vi "Examples.vi"(6 "Python version":string="3.9", 7 "Python":T1, 11 "Port":string) -> ()   [LabVIEW 2022 SP3]
uses:
  PythonCtrl.ctl
  Processors.ctl
panel:
  out "Python files":string[](array[string])
  in  "Location":bool
  in  "Folder":u16(ring) items=["home"]
  in  "Files":i32(listbox)
  in  "Code":string="Loading..."
  in  "Remove Button":bool
  in  "Paste":bool
  in  "Update":bool
  # "File Explorer\nversion 0"
  # "https://lego.github.io/MINDSTORMS-Robot-Inventor-hub-API/index.html"
  # "SPIKE Prime"
  # "Examples"
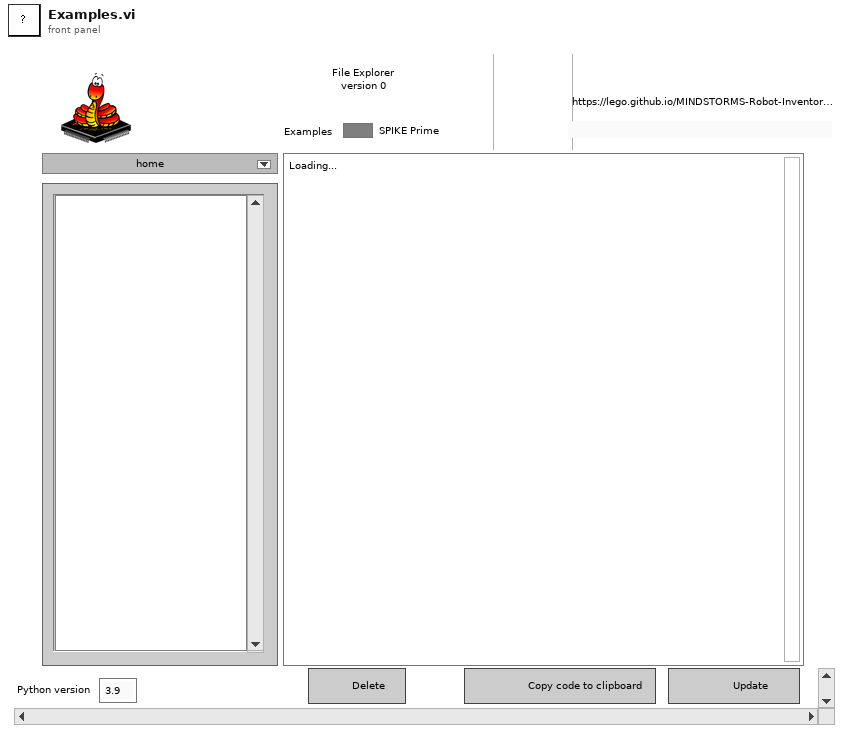
[diagram p1: front panel]
types:
  T1 = typedef "PythonCtrl.ctl" = cluster{"session":refnum<k35>, "PyPath":path, "Processor":T2, "Port":string, "version":string}
  T2 = typedef "Processors.ctl" = enum16{"SPIKE", "Pi", "Pi_ssh", "OpenMV", "Dunio"}
  T3 = enum16{"read", "write pause", "write port", "write path", "write all"}
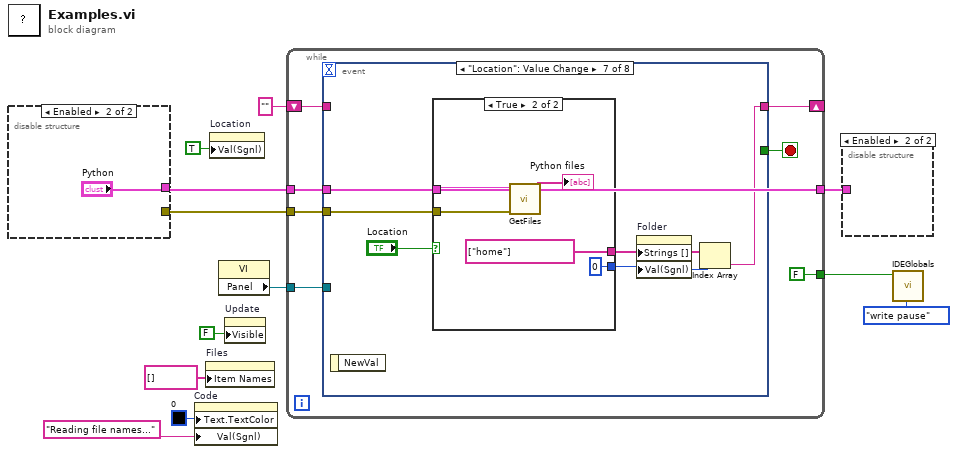
[diagram p0: block diagram]
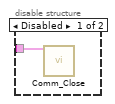
[diagram p2: hidden frame]
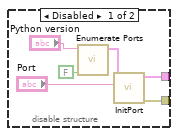
[diagram p3: hidden frame]
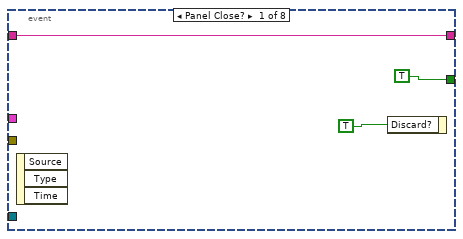
[diagram p4: hidden frame]
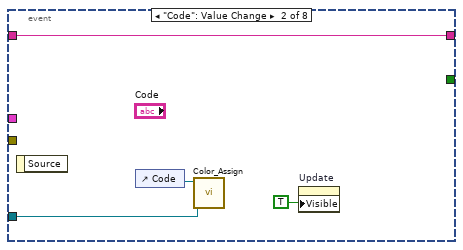
[diagram p5: hidden frame]
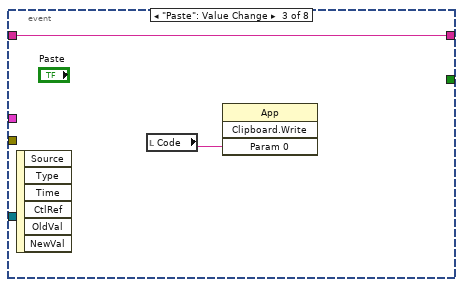
[diagram p6: hidden frame]
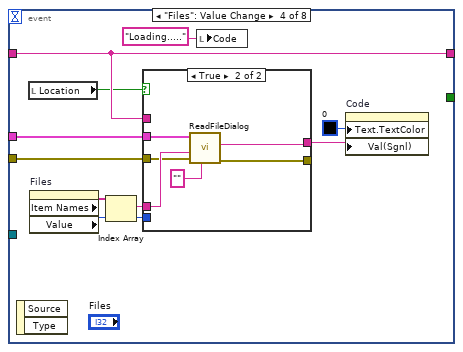
[diagram p7: hidden frame]
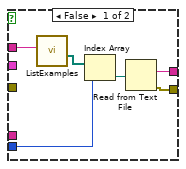
[diagram p8: hidden frame]
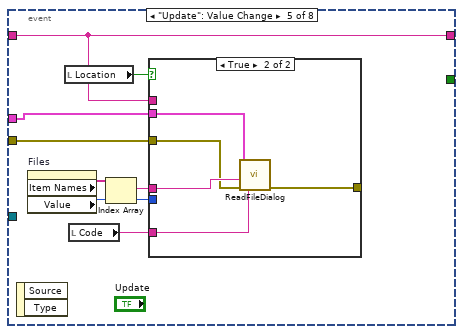
[diagram p9: hidden frame]
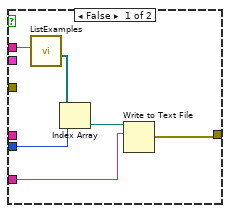
[diagram p10: hidden frame]
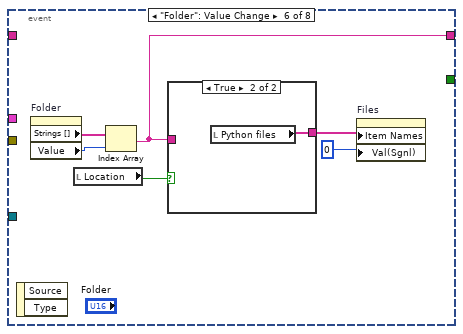
[diagram p11: hidden frame]
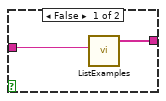
[diagram p12: hidden frame]
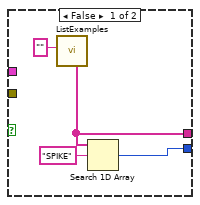
[diagram p13: hidden frame]
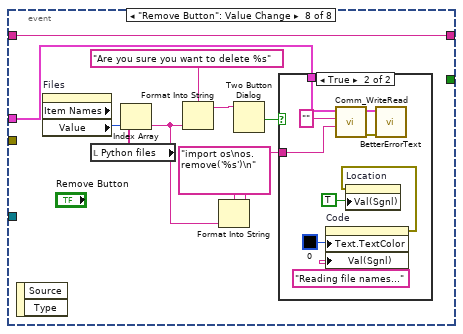
[diagram p14: hidden frame]
diagram:
  n1 = disable-structure shown="Enabled" {
    disable-tunnel: [w18 _] -> w7
    disable-tunnel: [w17 "Python"] -> w6
    frame Disabled {
      n2 = call "Enumerate Ports.vi"("list?"=FALSE, "Python version"="Python version") -> ("Python"=w15:T1)  [unwired: 4 in, 5 out]
      n3 = call "InitPort.vi"("Port"="Port", "Python"=w15) -> ("error out"=w18:errorcluster, "Python out"=w17:T1)  [unwired: 7 in, 1 out]
    }
    frame Enabled {
    }
  }
  n4 = property on="Code" class="Str"("Text.TextColor"=u32 0 ("Text.Text Colors:Text Color"), "Val(Sgnl)"="Reading file names...") -> ()  [unwired: 2 in, 2 out]
  n5 = property on="Files" class="LstBox (strict)"("Item Names"=string[] []) -> ()  [unwired: 2 in, 2 out]
  n6 = property on="Location" class="Bool (strict)"("Val(Sgnl)"=TRUE ("Value (Signaling)")) -> ()  [unwired: 2 in, 2 out]
  n7 = property class="VI"() -> ("Panel"=w12:refnum<vi>)  [unwired: 2 in, 2 out]
  n8 = property on="Update" class="Bool"("Visible"=FALSE) -> ()  [unwired: 2 in, 2 out]
  n9 = while {
    tunnel: w12 -> [w25]
    shift-right: [w24] -> _
    shift-left: "" ("Folder") -> [w23]
    tunnel: w6 -> [w20]
    tunnel: [FALSE ("pause?")] -> w1
    tunnel: w7 -> [w21]
    tunnel: [w20] -> w5
    stop <- w26 stop-if-true
    n10 = event shown="[6] \"Location\": Value Change" {
      selector: _ -> [_ _ _ _ _ _ _ _]
      dyn-events: _ -> [_ _ _ _ _ _ _ _]
      timeout: _ -> [_ _ _ _ _ _ _ _]
      tunnel: [TRUE ("stop") _ _ _ _ _ _ _] -> w26
      tunnel: w25 -> [_ w31 _ _ _ _ _ _]
      tunnel: [w27 w33 w35 w45 w65 w78 w89 w110] -> w24
      tunnel: w23 -> [w27 w33 w35 w45 w65 _ _ w110]
      tunnel: w20 -> [_ _ _ w43 w63 _ w91 w104]
      tunnel: w21 -> [_ _ _ w38 w58 _ w86 _]
      event Panel Close? {
        n11 = event-data() -> ()  [unwired: 1 in, 3 out]
        n12 = event-data("Discard?"=TRUE ("stop")) -> ()  [unwired: 1 in, 1 out]
      }
      event "Code": Value Change {
        n13 = event-data() -> ()  [unwired: 1 in, 1 out]
        n14 = control-ref of="Code"() -> (w30:refnum<vi>)
        n15 = call "Color_Assign.vi"("Front Panel"=w31, "Code"=w30) -> ()  [unwired: 9 in, 1 out]
        n16 = property on="Update" class="Bool"("Visible"=TRUE) -> ()  [unwired: 2 in, 2 out]
      }
      event "Paste": Value Change {
        n17 = event-data() -> ()  [unwired: 1 in, 6 out]
        n18 = local read "Code"() -> (w34:string)
        n19 = invoke class="App" method="Clipboard.Write"("Param 0"=w34) -> ()  [unwired: 3 in, 4 out]
      }
      event "Files": Value Change {
        n20 = event-data() -> ()  [unwired: 1 in, 2 out]
        n21 = local read "Location"() -> (w44:bool)
        n22 = property on="Files" class="LstBox (strict)"() -> ("Item Names"=w42:string[], "Value"=w40:i32)  [unwired: 2 in, 2 out]
        n23 = Index Array(array=w42, index=w40) -> (element=w41:string)
        n24 = case shown="True" w44 {
          tunnel: [w49 w56] -> w37
          tunnel: w45 -> [w48 _]
          tunnel: [w47 w55] -> _
          tunnel: w43 -> [_ w52]
          tunnel: w41 -> [_ w54]
          tunnel: w40 -> [w46 _]
          tunnel: w38 -> [_ w53]
          frame False {
            n25 = call "ListExamples.vi"("Folder"=w48) -> ("Paths"=w51:path[])  [unwired: 6 in, 4 out]
            n26 = Index Array(array=w51, index=w46) -> (element=w50:path)
            n27 = Read from Text File(file (use dialog)=w50) -> (text=w49:string, error out=w47:errorcluster)  [unwired: 3 in, 2 out]
          }
          frame True {
            n28 = call "ReadFileDialog.vi"("File Text"="" ("Folder"), "error in (no error)"=w53, "File name"=w54, "Python in"=w52) -> ("error out"=w55:errorcluster, "Console"=w56:string)  [unwired: 6 in]
          }
        }
        n29 = local write "Code"("Loading....." ("Folder")) -> ()
        n30 = property on="Code" class="Str"("Text.TextColor"=u32 0 ("Text.Text Colors:Text Color"), "Val(Sgnl)"=w37) -> ()  [unwired: 2 in, 2 out]
      }
      event "Update": Value Change {
        n31 = event-data() -> ()  [unwired: 1 in, 2 out]
        n32 = property on="Files" class="LstBox (strict)"() -> ("Item Names"=w62:string[], "Value"=w60:i32)  [unwired: 2 in, 2 out]
        n33 = local read "Location"() -> (w64:bool)
        n34 = local read "Code"() -> (w59:string)
        n35 = Index Array(array=w62, index=w60) -> (element=w61:string)
        n36 = case shown="True" w64 {
          tunnel: w65 -> [w69 _]
          tunnel: [w68 w76] -> _
          tunnel: w63 -> [_ w73]
          tunnel: w61 -> [_ w75]
          tunnel: w60 -> [w67 _]
          tunnel: w59 -> [w66 w74]
          tunnel: w58 -> [_ w72]
          frame False {
            n37 = call "ListExamples.vi"("Folder"=w69) -> ("Paths"=w71:path[])  [unwired: 6 in, 4 out]
            n38 = Index Array(array=w71, index=w67) -> (element=w70:path)
            n39 = Write to Text File(file (use dialog)=w70, text=w66) -> (error out=w68:errorcluster)  [unwired: 2 in, 2 out]
          }
          frame True {
            n40 = call "ReadFileDialog.vi"("File Text"=w74, "error in (no error)"=w72, "File name"=w75, "Python in"=w73) -> ("error out"=w76:errorcluster)  [unwired: 6 in, 1 out]
          }
        }
      }
      event "Folder": Value Change {
        n41 = event-data() -> ()  [unwired: 1 in, 2 out]
        n42 = property on="Folder" class="Ring (strict)"() -> ("Strings []"=w82:string[], "Value"=w81:u16)  [unwired: 2 in, 2 out]
        n43 = local read "Location"() -> (w77:bool)
        n44 = Index Array(array=w82, index=w81) -> (element=w78:string)
        n45 = case shown="True" w77 {
          tunnel: [w84 w85] -> w80
          tunnel: w78 -> [w83 _]
          frame False {
            n46 = call "ListExamples.vi"("Folder"=w83) -> ("filenames"=w84:string[])  [unwired: 6 in, 4 out]
          }
          frame True {
            n47 = local read "Python files"() -> (w85:string[])
          }
        }
        n48 = property on="Files" class="LstBox (strict)"("Item Names"=w80, "Val(Sgnl)"=u16 0 ("Value (Signaling)")) -> ()  [unwired: 2 in, 2 out]
      }
      event "Location": Value Change {
        n49 = event-data() -> ()  [unwired: 1 in, 1 out]
        n50 = case shown="True" "Location" {
          tunnel: w91 -> [_ w96]
          tunnel: [w94 string[] ["home"] ("folder names")] -> w88
          tunnel: [w92 u16 0 ("Value (Signaling)")] -> w87
          tunnel: w86 -> [_ w97]
          frame False {
            n51 = call "ListExamples.vi"("Folder"="") -> ("folder names"=w94:string[])  [unwired: 6 in, 4 out]
            n52 = Search 1D Array(1D array=w94, element="SPIKE") -> (index of element=w92:i32)  [unwired: 1 in]
          }
          frame True {
            n53 = call "GetFiles.vi"("error in (no error)"=w97, "Python"=w96) -> ("all files"=→"Python files":string[])  [unwired: 8 in, 1 out]
          }
        }
        n54 = property on="Folder" class="Ring (strict)"("Strings []"=w88, "Val(Sgnl)"=w87) -> ()  [unwired: 2 in, 2 out]
        n55 = Index Array(array=w88, index=w87) -> (element=w89:string)
      }
      event "Remove Button": Value Change {
        n56 = event-data() -> ()  [unwired: 1 in, 2 out]
        n57 = property on="Files" class="LstBox (strict)" props=["Item Names", "Value"]() -> ("Value"=w109:i32)  [unwired: 2 in, 3 out]
        n58 = local read "Python files"() -> (w106:string[])
        n59 = Index Array(array=w106, index=w109) -> (element=w103:string)
        n60 = Format Into String(format string="Are you sure you want to delete %s", w103) -> (resulting string=w107:string)  [unwired: 2 in, 1 out]
        n61 = Format Into String(format string="import os\nos.remove('%s')\n" ("regular expression"), w103) -> (resulting string=w101:string)  [unwired: 2 in, 1 out]
        n62 = Two Button Dialog(message=w107) -> (T button?=w105:bool)  [unwired: 2 in]
        n63 = case shown="True" w105 {
          tunnel: w104 -> [_ w116]
          tunnel: w101 -> [_ w115]
          frame False {
          }
          frame True {
            n64 = property on="Code" class="Str"("Text.TextColor"=u32 0 ("Text.Text Colors:Text Color"), "Val(Sgnl)"="Reading file names...") -> (error out=w111:errorcluster)  [unwired: 2 in, 1 out]
            n65 = call "Comm_WriteRead.vi"("Code"=w115, "Console In"="" ("Text to write"), "Python"=w116) -> ("error out"=w118:errorcluster, "Python"=w119:T1)  [unwired: 6 in, 1 out]
            n66 = property on="Location" class="Bool (strict)"(error in=w111, "Val(Sgnl)"=TRUE ("Value (Signaling)")) -> ()  [unwired: 1 in, 2 out]
            n67 = call "BetterErrorText.vi"("error in (no error)"=w118, "Python"=w119) -> ()  [unwired: 8 in, 2 out]
          }
        }
      }
    }
  }
  n68 = disable-structure shown="Enabled" {
    disable-tunnel: w5 -> [w120 _]
    frame Disabled {
      n69 = call "Comm_Close.vi"("Python in"=w120) -> ()  [unwired: 9 in, 2 out]
    }
    frame Enabled {
    }
  }
  n70 = call "IDEGlobals.vi"("task"=T3."write pause", "pause?"=w1) -> ()  [unwired: 7 in, 3 out]
